vi "Convert_String_to_TimeStamp.vi"(1 "date/time string":string) -> (0 "Resulting Time Stamp":timestamp format="%<%I:%M:%S %p\n%x>T")   [LabVIEW 2011]
doc: "This VI convert a date/time string back to a time stamp."
panel:
  # "This control should have data in the form:\n4/30/2004 7:48:47 PM"
  # "3/29/2008 12:00:07 AM"
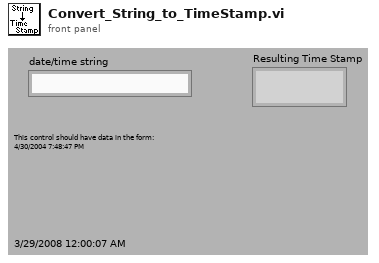
[diagram p1: front panel]
types:
  T1 = cluster{"second":i32, "minute":i32, "hour":i32, "day of month":i32, "month":i32, "year":i32, "day of week":i32, "day of year":i32, "is DST":i32}
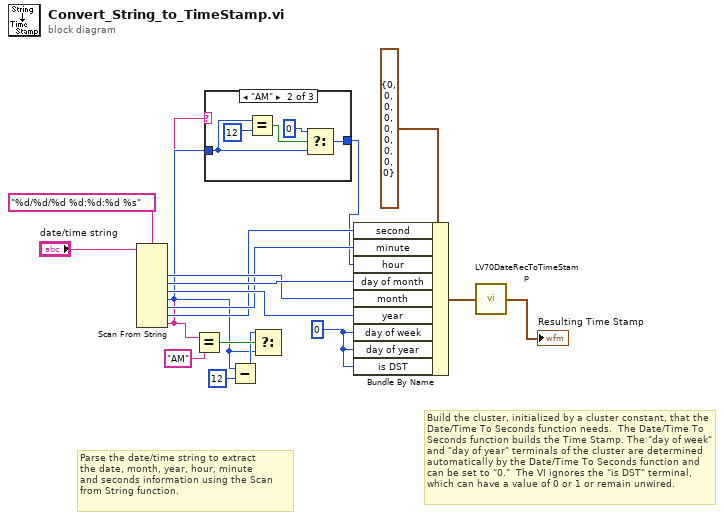
[diagram p0: block diagram]
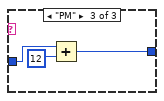
[diagram p3: hidden frame]
diagram:
  w6 = 0
  # "Build the cluster, initialized by a cluster constant, that the Date/Time To Seconds function needs.  The Date/Time To Seconds function builds the Time Stamp. The \"day of week\" and \"day of year\" terminals of the cluster are determined automatically by the Date/Time To Seconds function and can be set to \"0.\"  The VI ignores the \"is DST\" terminal, which can have a value of 0 or 1 or remain unwired."
  # "Parse the date/time string to extract \nthe date, month, year, hour, minute \nand seconds information using the Scan\nfrom String function."
  n1 = Scan From String(format string="%d/%d/%d %d:%d:%d %s", input string="date/time string") -> (output 1=w13:i32, output 2=w14:i32, output 3=w12:i32, output 4=w3:i32, output 5=w11:i32, output 6=w10:i32, output 7=w1:string)  [unwired: 9 in, 3 out]
  n2 = Equal?(x=w1, y="AM") -> (x = y?=w5:bool)
  n3 = case shown="\"AM\"" w1 {
    tunnel: w3 -> [w19 w22 w26]
    tunnel: [w19 w20 w25] -> w2
    frame Default {
    }
    frame "AM" {
      n4 = Equal?(x=w22, y=12) -> (x = y?=w23:bool)
      n5 = Select(t=0, s=w23, f=w22) -> (s? t:f=w20:i32)
    }
    frame "PM" {
      n6 = Add(x=w26, y=12) -> (x+y=w25:i32)
    }
  }
  n7 = Subtract(x=w3, y=12) -> (x-y=w4:i32)
  n8 = Select(t=w4, s=w5, f=w3) -> ()  [unwired: 1 out]
  n9 = Bundle By Name(cluster=T1 {"second"=0, "minute"=0, "hour"=0, "day of month"=0, "month"=0, "year"=0, "day of week"=0, "day of year"=0, "is DST"=0} ("date time rec"), "second"=w10, "minute"=w11, "hour"=w2, "day of month"=w14, "month"=w13, "year"=w12, "day of week"=w6, "day of year"=w6, "is DST"=w6) -> (w7:T1)
  n10 = call <vilib>:"LV70DateRecToTimeStamp.vi"("date time rec"=w7) -> ("Time Stamp"=→"Resulting Time Stamp":timestamp)
